vi "2LOOPs-DAQ.vi"() -> ()   [LabVIEW 2021]
panel:
  out "Chart":dbl(graph)
  in  "PauseDAQ":bool
  in  "StartDAQ":bool
  out "ErrO":errorcluster
  in  "ErrI":errorcluster
  in  "Exit":bool
  # "Messages will be sent\nto DAQ Loop to contol\nthe DAQ Start / Pause."
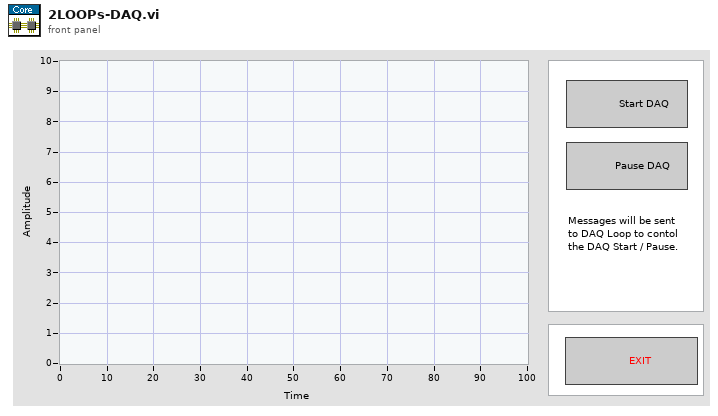
[diagram p1: front panel]
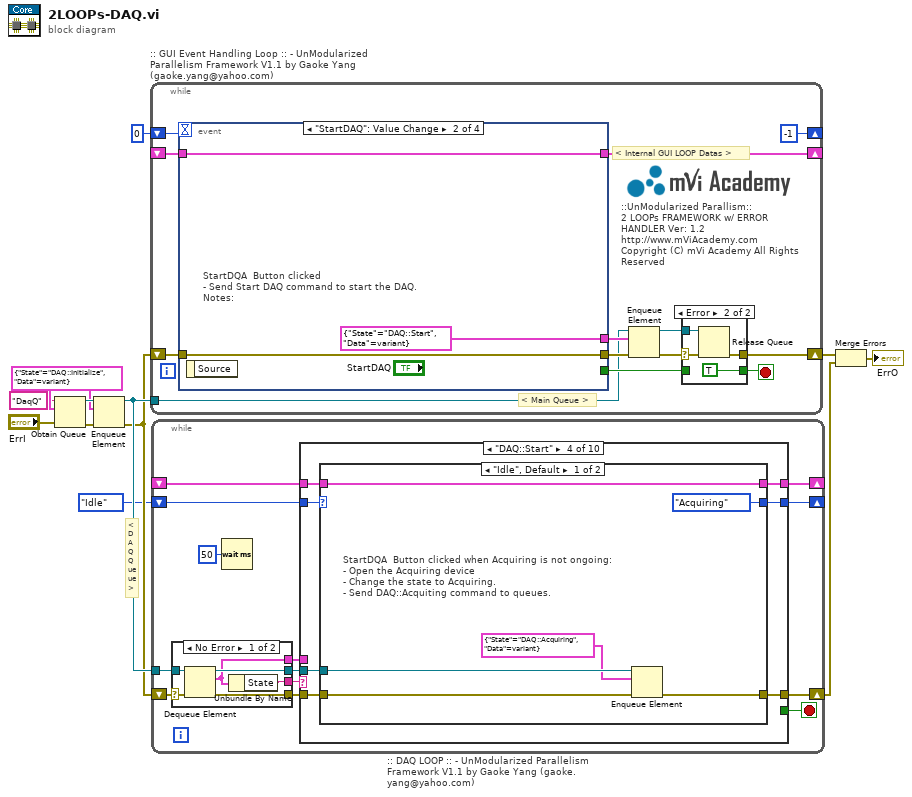
[diagram p0: block diagram]
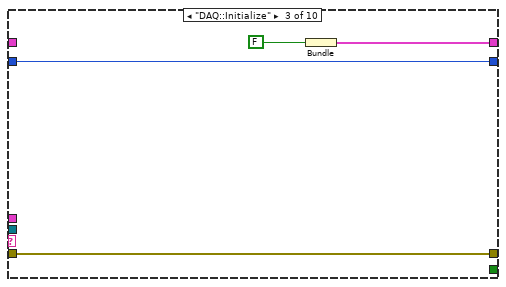
[diagram p4: hidden frame]
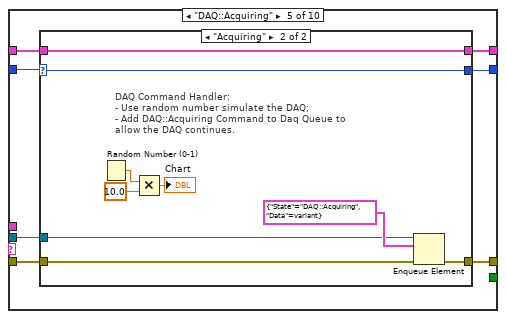
[diagram p6: hidden frame]
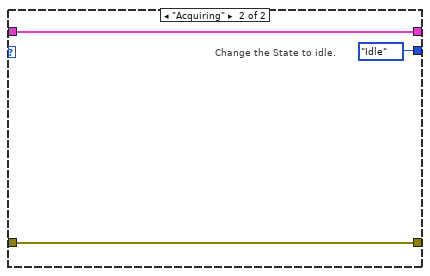
[diagram p9: hidden frame]
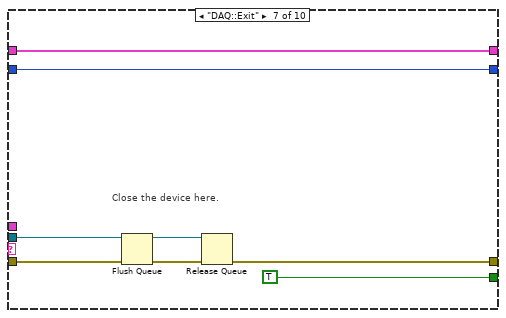
[diagram p10: hidden frame]
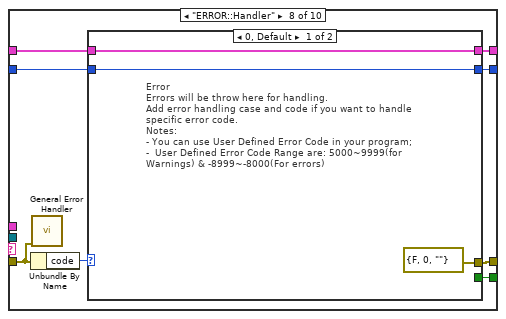
[diagram p11: hidden frame]
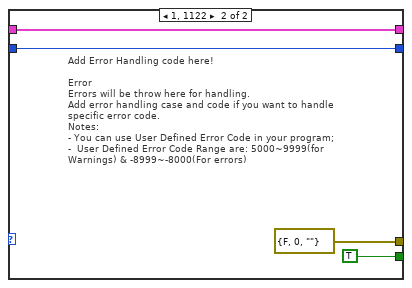
[diagram p12: hidden frame]
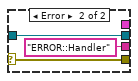
[diagram p15: hidden frame]
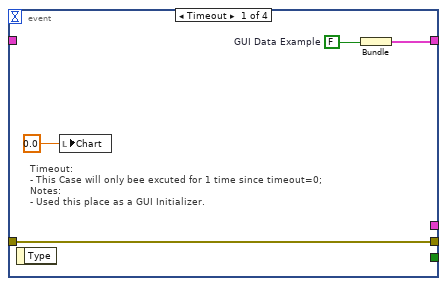
[diagram p17: hidden frame]
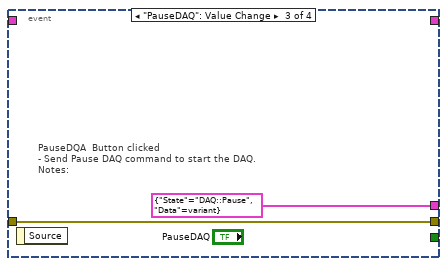
[diagram p18: hidden frame]
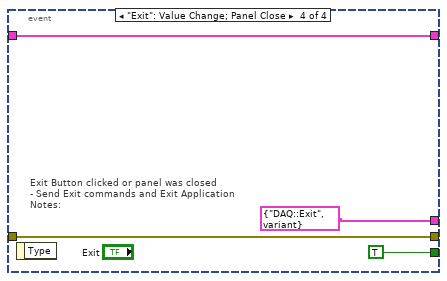
[diagram p19: hidden frame]
diagram:
  w8 = cluster{"State":string, "Data":variant} {"State"="DAQ::Initialize", "Data"=variant} ("MainQueue")
  # "< DAQ Queue >"
  n1 = Obtain Queue(name (unnamed)="DaqQ", element data type=w8, error in (no error)="ErrI") -> (queue out=w10:refnum<queue>, error out=w9:errorcluster)  [unwired: 2 in, 1 out]
  n2 = Enqueue Element(queue=w10, element=w8, error in (no error)=w9) -> (queue out=w6:refnum<queue>, error out=w5:errorcluster)  [unwired: 2 out]
  n3 = while ":: GUI Event Handling Loop :: - UnModularized Parallelism Framework V1.1 by Gaoke Yang (gaoke.yang@yahoo.com)" {
    tunnel: w6 -> [w15]
    shift-right: [w24] -> w12
    shift-left: w5 -> [w25]
    shift-right: [-1] -> _
    shift-left: 0 -> [w22]
    shift-right: [w21] -> _
    shift-left: _ -> [w20]
    stop <- w18 stop-if-true
    # "::UnModularized Parallism::\n2 LOOPs FRAMEWORK w/ ERROR HANDLER Ver: 1.2\nhttp://www.mViAcademy.com\nCopyright (C) mVi Academy All Rights Reserved"
    # "< Internal GUI LOOP Datas >"
    # "< Main Queue >"
    n4 = event shown="[1] \"StartDAQ\": Value Change" {
      selector: _ -> [_ _ _ _]
      dyn-events: _ -> [_ _ _ _]
      timeout: w22 -> [_ _ _ _]
      tunnel: [_ _ _ TRUE ("Exit")] -> w19
      tunnel: w25 -> [w35 w38 w40 w41]
      tunnel: [w35 w38 w40 w41] -> w17
      tunnel: [_ cluster{"State":string, "Data":variant} {"State"="DAQ::Start", "Data"=variant} ("MainQueue") cluster{"State":string, "Data":variant} {"State"="DAQ::Pause", "Data"=variant} ("MainQueue") cluster{"State":string, "Data":variant} {"State"="DAQ::Exit", "Data"=variant} ("Packet")] -> w16
      tunnel: [w33 w37 _ w44] -> w21
      tunnel: w20 -> [_ w37 _ w44]
      event Timeout {
        w34 = FALSE  # GUI Data Example
        # "Timeout:\n- This Case will only bee excuted for 1 time since timeout=0;\nNotes:\n- Used this place as a GUI Initializer."
        n5 = event-data() -> ()  [unwired: 2 out]
        n6 = local write "Chart"(0.0 ("Chart")) -> ()
        n7 = Bundle("GUI Data Example"=w34) -> (w33:cluster{"GUI Data Example":bool})  [unwired: 1 in]
      }
      event "StartDAQ": Value Change {
        # "StartDQA  Button clicked\n- Send Start DAQ command to start the DAQ.\nNotes:"
        n8 = event-data() -> ()  [unwired: 2 out]
      }
      event "PauseDAQ": Value Change {
        # "PauseDQA  Button clicked\n- Send Pause DAQ command to start the DAQ.\nNotes:"
        n9 = event-data() -> ()  [unwired: 2 out]
      }
      event "Exit": Value Change; Panel Close {
        # "Exit Button clicked or panel was closed\n- Send Exit commands and Exit Application\nNotes:"
        n10 = event-data() -> ()  [unwired: 2 out]
      }
    }
    n11 = Enqueue Element(queue=w15, element=w16, error in (no error)=w17) -> (queue out=w13:refnum<queue>, error out=w14:errorcluster)  [unwired: 2 out]
    n12 = case shown="Error" w14 {
      selector: w14 -> [w27 w30]
      tunnel: [w27 w28] -> w24
      tunnel: w19 -> [w26 _]
      tunnel: [w26 TRUE ("Exit")] -> w18
      tunnel: w13 -> [_ w29]
      frame No Error {
      }
      frame Error {
        n13 = Release Queue(queue=w29, error in (no error)=w30) -> (error out=w28:errorcluster)  [unwired: 1 in, 2 out]
      }
    }
  }
  n14 = while ":: DAQ LOOP :: - UnModularized Parallelism Framework V1.1 by Gaoke Yang (gaoke.yang@yahoo.com)" {
    tunnel: w6 -> [w57]
    shift-right: [w51] -> w4
    shift-left: w5 -> [w56]
    shift-right: [w48] -> _
    shift-left: _ -> [w49]
    shift-right: [w45] -> _
    shift-left: enum16{"Idle", "Acquiring"}."Idle" -> [w46]
    stop <- w50 stop-if-true
    n15 = case shown="No Error" w56 {
      selector: w56 -> [w144 w152]
      tunnel: w57 -> [w149 w150]
      tunnel: [w148 w152] -> w55
      tunnel: [w147 w150] -> w53
      tunnel: [w146 "ERROR::Handler" ("State")] -> w54
      tunnel: [w145 _] -> w52
      frame No Error {
        n16 = Dequeue Element(queue=w149, error in (no error)=w144) -> (queue out=w147:refnum<queue>, element=w145:cluster{"State":string, "Data":variant}, error out=w148:errorcluster)  [unwired: 2 out]
        n17 = Unbundle By Name(w145) -> ("State"=w146:string)
      }
      frame Error {
      }
    }
    n18 = Wait (ms)(milliseconds to wait=u32 50) -> ()  [unwired: 1 out]
    n19 = case shown="\"DAQ::Start\"" w54 {
      tunnel: w55 -> [w59 w63 w65 w73 w89 w104 w121 w126 w140 w143]
      tunnel: [w59 w63 w65 w74 w90 w103 w118 w128 w140 w143] -> w51
      tunnel: [_ _ _ _ _ _ TRUE w127 _ _] -> w50
      tunnel: w53 -> [_ _ _ w72 w88 _ w120 _ _ _]
      tunnel: [w60 w62 w66 w71 w86 w106 w116 w129 w139 w142] -> w48
      tunnel: w49 -> [w60 w62 _ w70 w87 w107 w116 w130 w139 w142]
      tunnel: w52 -> [_ _ _ _ _ _ _ _ _ _]
      tunnel: w46 -> [w58 w61 w64 w69 w85 w105 w115 w124 w138 w141]
      tunnel: [w58 w61 w64 w68 w84 w108 w115 w123 w138 w141] -> w45
      frame "IDLE", Default {
      }
      frame "-------- DAQ ---------" {
      }
      frame "DAQ::Initialize" {
        n20 = Bundle(FALSE) -> (w66:cluster{bool})  [unwired: 1 in]
      }
      frame "DAQ::Start" {
        n21 = case shown="\"Idle\", Default" w69 {
          selector: w69 -> [_ w81]
          tunnel: [w80 w82] -> w74
          tunnel: w73 -> [w79 w82]
          tunnel: w72 -> [w78 _]
          tunnel: [w76 w83] -> w71
          tunnel: w70 -> [w76 w83]
          tunnel: [enum16{"Idle", "Acquiring"}."Acquiring" w81] -> w68
          frame "Idle", Default {
            # "StartDQA  Button clicked when Acquiring is not ongoing:\n- Open the Acquiring device\n- Change the state to Acquiring.\n- Send DAQ::Acquiting command to queues."
            n22 = Enqueue Element(queue=w78, element=cluster{"State":string, "Data":variant} {"State"="DAQ::Acquiring", "Data"=variant} ("DaqQueue"), error in (no error)=w79) -> (error out=w80:errorcluster)  [unwired: 3 out]
          }
          frame "Acquiring" {
            # "The system is already acquiring. \nIgnore the \"Start\" message."
          }
        }
      }
      frame "DAQ::Acquiring" {
        n23 = case shown="\"Acquiring\"" w85 {
          selector: w85 -> [w92 w94]
          tunnel: [w91 w102] -> w90
          tunnel: w89 -> [w91 w101]
          tunnel: w88 -> [_ w99]
          tunnel: w87 -> [w93 w95]
          tunnel: [w93 w95] -> w86
          tunnel: [w92 w94] -> w84
          frame "Idle", Default {
            # "Ignore \"Acquire\" command when the acquisition is idle."
          }
          frame "Acquiring" {
            # "DAQ Command Handler: \n- Use random number simulate the DAQ;\n- Add DAQ::Acquiring Command to Daq Queue to allow the DAQ continues."
            n24 = Random Number (0-1)() -> (number: 0 to 1=w98:dbl)
            n25 = Multiply(x=w98, y=10.0) -> (x*y=→"Chart":dbl)
            n26 = Enqueue Element(queue=w99, element=cluster{"State":string, "Data":variant} {"State"="DAQ::Acquiring", "Data"=variant} ("DaqQueue"), error in (no error)=w101) -> (error out=w102:errorcluster)  [unwired: 3 out]
          }
        }
      }
      frame "DAQ::Pause" {
        n27 = case shown="\"Idle\", Default" w105 {
          selector: w105 -> [w110 _]
          tunnel: [w110 enum16{"Idle", "Acquiring"}."Idle"] -> w108
          tunnel: w107 -> [w111 w113]
          tunnel: [w111 w113] -> w106
          tunnel: w104 -> [w109 w112]
          tunnel: [w109 w112] -> w103
          frame "Idle", Default {
            # "Already idle, ignore Pause command."
          }
          frame "Acquiring" {
            # "Change the State to idle."
          }
        }
      }
      frame "DAQ::Exit" {
        # "Close the device here."
        n28 = Flush Queue(queue=w120, error in (no error)=w121) -> (queue out=w117:refnum<queue>, error out=w119:errorcluster)  [unwired: 1 out]
        n29 = Release Queue(queue=w117, error in (no error)=w119) -> (error out=w118:errorcluster)  [unwired: 1 in, 2 out]
      }
      frame "ERROR::Handler" {
        n30 = Unbundle By Name(w126) -> ("code"=w125:i32)
        n31 = call <vilib>:"General Error Handler.vi"("error in (no error)"=w126) -> ()  [unwired: 10 in, 5 out]
        n32 = case shown="0, Default" w125 {
          tunnel: [w133 w137] -> w129
          tunnel: w130 -> [w133 w137]
          tunnel: [errorcluster {"status"=FALSE, "code"=0, "source"=""} ("error out") errorcluster {"status"=FALSE, "code"=0, "source"=""} ("error out")] -> w128
          tunnel: [_ TRUE] -> w127
          tunnel: w124 -> [w131 w134]
          tunnel: [w131 w134] -> w123
          frame 0, Default {
            # "Error\nErrors will be throw here for handling.\nAdd error handling case and code if you want to handle specific error code.\nNotes:\n- You can use User Defined Error Code in your program;\n-  User Defined Error Code Range are: 5000~9999(for Warnings) & -8999~-8000(For errors)"
          }
          frame 1, 1122 {
            # "Add Error Handling code here!\n\nError\nErrors will be throw here for handling.\nAdd error handling case and code if you want to handle specific error code.\nNotes:\n- You can use User Defined Error Code in your program;\n-  User Defined Error Code Range are: 5000~9999(for Warnings) & -8999~-8000(For errors)"
          }
        }
      }
      frame "----- User Case ------" {
      }
      frame "Reserved" {
      }
    }
  }
  n33 = Merge Errors(w12, w4) -> (→"ErrO":errorcluster)
